vi "Register gRPC Methods.vi"(8 "error in (no error)":errorcluster, 11 "OOP Server in":refnum<class "OOP Server.lvclass">) -> (0 "error out":errorcluster, 3 "OOP Server out":refnum<class "OOP Server.lvclass">)   [LabVIEW 2019, in "OOP Server.lvlib" / "OOP Server.lvclass"]
uses:
  OOP Server.lvclass
  typeDefs/Server gRPC UEs.ctl
  gRPC interface/Server API/typeDefs/gRPCId Cluster UE.ctl
  gRPC interface/Server API/typeDefs/gRPCId Cluster.ctl
  gRPC interface/Server API/typeDefs/grpcId.ctl
  typeDefs/Server Internal UEs.ctl
  typeDefs/Server Internal Data.ctl
  OOP Server.lvclass/OOP Server.ctl
  gRPC interface/gprc-lvsupport.lvlib
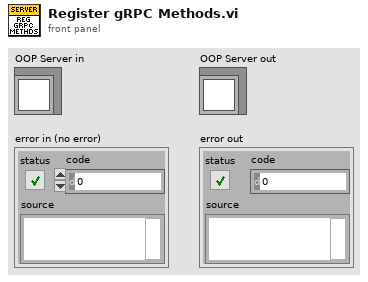
[diagram p1: front panel]
types:
  T1 = typedef "OOP Server.lvlib/OOP Server.lvclass/Server Internal UEs.ctl" = cluster{"Invoke Internal UE":refnum<user-event>, "Query Internal UE":refnum<user-event>, "Register Internal UE":refnum<user-event>}
  T2 = typedef "OOP Server.lvlib/OOP Server.lvclass/Server gRPC UEs.ctl" = cluster{"Invoke gRPC UEs":T3, "Query gRPC UEs":T3, "Register gRPC UEs":T3}
  T3 = typedef "gprc-lvsupport.lvlib/gRPCId Cluster UE.ctl" = refnum<user-event>
  T4 = typedef "gprc-lvsupport.lvlib/grpcId.ctl" = u64
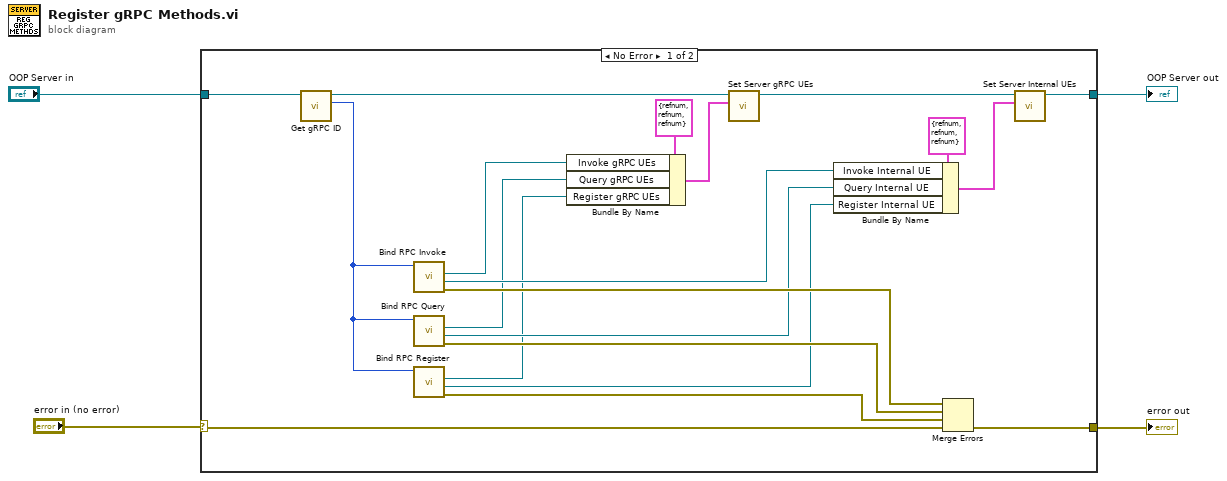
[diagram p0: block diagram]
diagram:
  n1 = case shown="No Error" "error in (no error)" {
    selector: "error in (no error)" -> [w5 w25]
    tunnel: "OOP Server in" -> [w22 w26]
    tunnel: [w21 w25] -> w3
    tunnel: [w17 w26] -> w2
    frame No Error {
      n2 = call "Get gRPC ID.vi"("OOP Server in"=w22) -> ("gRPC ID"=w24:T4, "OOP Server out"=w23:refnum<class "OOP Server.lvclass">)  [unwired: 9 in]
      n3 = call "Bind RPC Invoke.vi"("gRPCid server in"=w24) -> ("error out"=w18:errorcluster, "Invoke Internal UE"=w13:refnum<user-event>, "Invoke gRPC UE"=w8:refnum<user-event>)  [unwired: 7 in, 1 out]
      n4 = call "Bind RPC Query.vi"("gRPCid server in"=w24) -> ("error out"=w19:errorcluster, "Query Internal UE"=w14:refnum<user-event>, "Query gRPC UE"=w7:refnum<user-event>)  [unwired: 7 in, 1 out]
      n5 = call "Bind RPC Register.vi"("gRPCid server in"=w24) -> ("error out"=w20:errorcluster, "Register Internal UE"=w15:refnum<user-event>, "Register gRPC UE"=w9:refnum<user-event>)  [unwired: 7 in, 1 out]
      n6 = Bundle By Name(cluster=T2 {"Invoke gRPC UEs"=refnum, "Query gRPC UEs"=refnum, "Register gRPC UEs"=refnum} ("gRPC Server Method Events"), "Invoke gRPC UEs"=w8, "Query gRPC UEs"=w7, "Register gRPC UEs"=w9) -> (w10:T2)
      n7 = call "Set Server gRPC UEs.vi"("Server gRPC UEs"=w10, "OOP Server in"=w23) -> ("OOP Server out"=w11:refnum<class "OOP Server.lvclass">)  [unwired: 9 in]
      n8 = Bundle By Name(cluster=T1 {"Invoke Internal UE"=refnum, "Query Internal UE"=refnum, "Register Internal UE"=refnum} ("Server Internal UEs"), "Invoke Internal UE"=w13, "Query Internal UE"=w14, "Register Internal UE"=w15) -> (w16:T1)
      n9 = Merge Errors(w18, w19, w20, w5) -> (w21:errorcluster)
      n10 = call "Set Server Internal UEs.vi"("Server Internal UEs"=w16, "OOP Server in"=w11) -> ("OOP Server out"=w17:refnum<class "OOP Server.lvclass">)  [unwired: 9 in]
    }
    frame Error {
    }
  }
  "error out" <- w3
  "OOP Server out" <- w2
